vi "Set Calculation Settings.vi"(7 "GUI Settings":T1, 8 "error in":errorcluster, 11 "Calculation Settings":T3={"Verbose"=FALSE, "Uncertainty Calculation Method"=enum."none", "Correlations"={"Required"=FALSE, "Generate"=TRUE}, "Degrees of Freedom"={"Required"=FALSE, "Generate"=FALSE}, "MCM Calculation Settings"={"Repeats"=100, "Verbose"=TRUE, "Parallelization method"=enum."Single Core", "Processors"=1, "Temporary directory"=".", "Randomize"=TRUE}} {"MCM Calculation Settings"."Processors" min=1 step=1; "MCM Calculation Settings"."Repeats" min=1 step=1}) -> (0 "error out":errorcluster)   [LabVIEW 2013]
uses:
  TD Calculation Settings.ctl
  TD Uncertainty Calculation Method.ctl
  TD Correlation Calculation Settings.ctl
  TD DOF Calculation Settings.ctl
  TD MCM Calculation Settings.ctl
  TD MCM Calculation Method.ctl
  TD GUI Settings.ctl
  TD GUI Engine.ctl
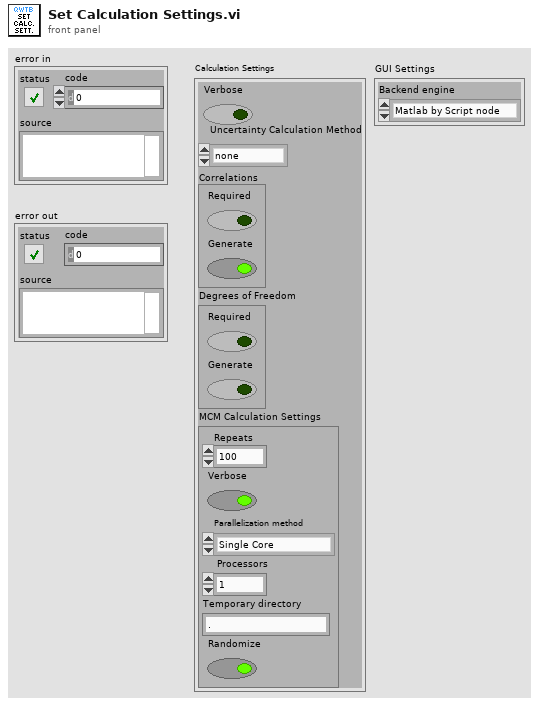
[diagram p1: front panel]
types:
  T1 = typedef "TD GUI Settings.ctl" = cluster{"Backend engine":T2}
  T2 = typedef "TD GUI Engine.ctl" = enum16{"Matlab by Script node", "GNU Octave by GOLPI"}
  T3 = typedef "TD Calculation Settings.ctl" = cluster{"Verbose":bool, "Uncertainty Calculation Method":T4, "Correlations":T5, "Degrees of Freedom":T6, "MCM Calculation Settings":T7}
  T4 = typedef "TD Uncertainty Calculation Method.ctl" = enum16{"none", "GUF", "MCM"}
  T5 = typedef "TD Correlation Calculation Settings.ctl" = cluster{"Required":bool, "Generate":bool}
  T6 = typedef "TD DOF Calculation Settings.ctl" = cluster{"Required":bool, "Generate":bool}
  T7 = typedef "TD MCM Calculation Settings.ctl" = cluster{"Repeats":i32, "Verbose":bool, "Parallelization method":T8, "Processors":i32, "Temporary directory":string, "Randomize":bool}
  T8 = typedef "TD MCM Calculation Method.ctl" = enum16{"Single Core", "Multi Core", "Multi Station"}
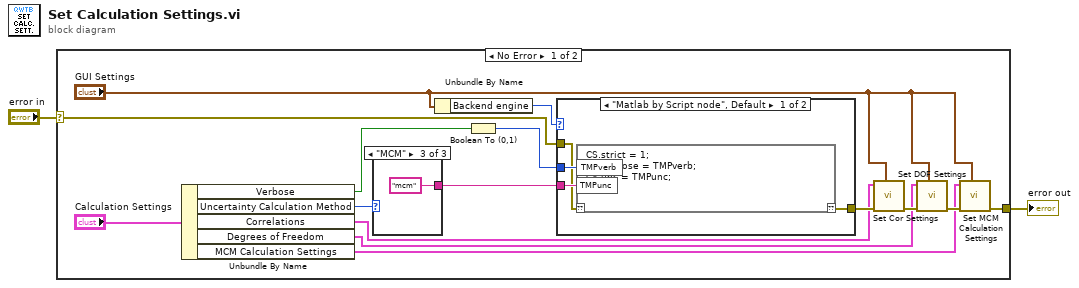
[diagram p0: block diagram]
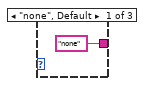
[diagram p3: hidden frame]
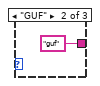
[diagram p4: hidden frame]
diagram:
  n1 = case shown="No Error" "error in" {
    selector: "error in" -> [w15 w26]
    tunnel: [w5 w26] -> w2
    frame No Error {
      n2 = Unbundle By Name("Calculation Settings") -> ("Verbose"=w12:bool, "Uncertainty Calculation Method"=w13:T4, "Correlations"=w9:T5, "Degrees of Freedom"=w7:T6, "MCM Calculation Settings"=w4:T7)
      n3 = case shown="\"MCM\"" w13 {
        tunnel: ["none" ("String") "guf" ("String") "mcm" ("String")] -> w16
        frame "none", Default {
        }
        frame "GUF" {
        }
        frame "MCM" {
        }
      }
      n4 = Unbundle By Name("GUI Settings") -> ("Backend engine"=w11:T2)
      n5 = Boolean To (0,1)(Boolean=w12) -> (0, 1=w17:i16)
      n6 = case shown="\"Matlab by Script node\", Default" w11 {
        tunnel: [w21 w22] -> w10
        tunnel: w17 -> [w20 _]
        tunnel: w16 -> [w19 _]
        tunnel: w15 -> [w18 w22]
        frame "Matlab by Script node", Default {
          n7 = script code="CS.strict = 1;\nCS.verbose = TMPverb;\nCS.unc = TMPunc;"("??"=w18, "TMPverb"=w20, "TMPunc"=w19) -> ("??"=w21:errorcluster)
        }
        frame "GNU Octave by GOLPI" {
          # "#2DO"
        }
      }
      n8 = call "Set Cor Settings.vi"("GUI Settings"="GUI Settings", "error in"=w10, "Correlations"=w9) -> ("error out"=w8:errorcluster)  [unwired: 8 in]
      n9 = call "Set DOF Settings.vi"("GUI Settings"="GUI Settings", "error in"=w8, "Degrees Of Freedom"=w7) -> ("error out"=w6:errorcluster)  [unwired: 8 in]
      n10 = call "Set MCM Calculation Settings.vi"("GUI Settings"="GUI Settings", "error in"=w6, "MCM Calcualtion Settings"=w4) -> ("error out"=w5:errorcluster)  [unwired: 8 in]
    }
    frame Error {
    }
  }
  "error out" <- w2
